vi "GetPSQL Datatype.vi"(8 "error in (no error)":errorcluster, 9 "Column":string, 10 "Table":string, 11 "LV-Data.PGSQL in":refnum<class "LV-Data.PGSQL.lvclass">) -> (2 "Get:Get String":string, 3 "LV-Data.PGSQL out":refnum<class "LV-Data.PGSQL.lvclass">)   [LabVIEW 2016]
uses:
  LV-Data.PGSQL.lvclass
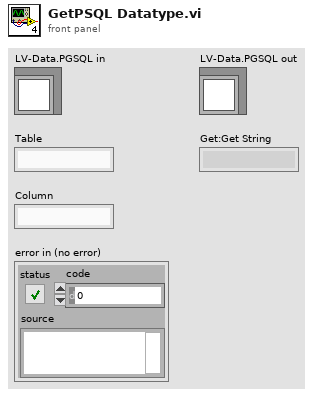
[diagram p1: front panel]
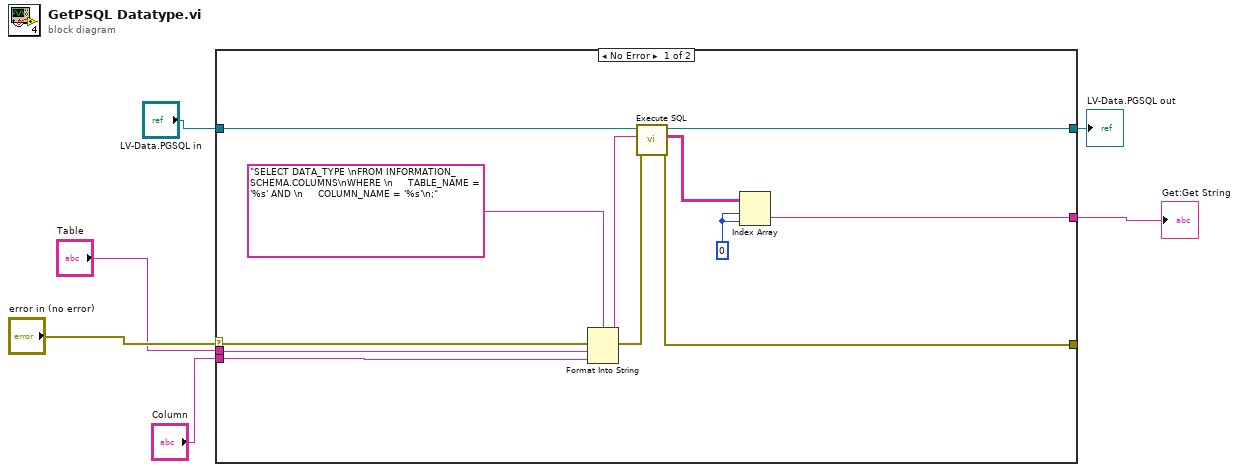
[diagram p0: block diagram]
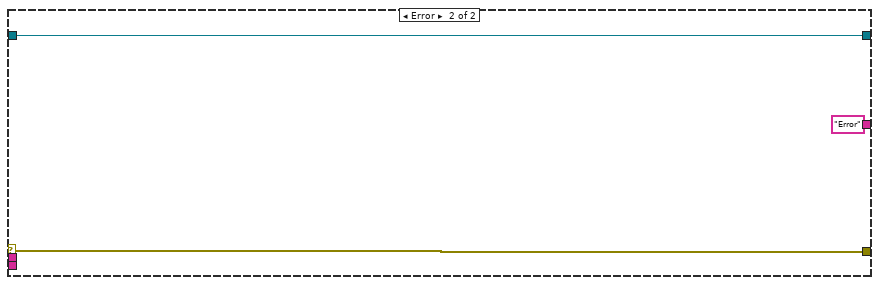
[diagram p2: hidden frame]
diagram:
  n1 = case shown="No Error" "error in (no error)" {
    selector: "error in (no error)" -> [w12 w21]
    tunnel: "Column" -> [w13 _]
    tunnel: [w10 w21] -> _
    tunnel: [w11 w19] -> w2
    tunnel: "Table" -> [w14 _]
    tunnel: [w9 "Error" ("Get:Get String")] -> w5
    tunnel: "LV-Data.PGSQL in" -> [w8 w19]
    frame No Error {
      w16 = 0 ("index (row)")
      n2 = Format Into String(format string="SELECT DATA_TYPE \nFROM INFORMATION_SCHEMA.COLUMNS\nWHERE \n     TABLE_NAME = '%s' AND \n     COLUMN_NAME = '%s'\n;", error in=w12, w14, w13) -> (resulting string=w7:string, error out=w15:errorcluster)  [unwired: 1 in]
      n3 = call "Execute SQL.vi"("error in"=w15, "SQL"=w7, "Data.PG"=w8) -> ("error out"=w10:errorcluster, "Result"=w18:string[][], "Data.PG out"=w11:refnum<class "LV-Data.PGSQL.lvclass">)  [unwired: 6 in]
      n4 = Index Array(array=w18, index (row)=w16, index (col)=w16) -> (element=w9:string)
    }
    frame Error {
    }
  }
  "Get:Get String" <- w5
  "LV-Data.PGSQL out" <- w2
